vi "Find All COM ports with device Attached.vi"(8 "Error In":errorcluster) -> (0 "Error Out":errorcluster, 3 "List of COM ports with something attached":string[](array[string]))   [LabVIEW 2014]
uses:
  <vilib>/Instr/_visa.llb/VISA Find Search Mode.ctl
panel:
  # "(COM)|?"
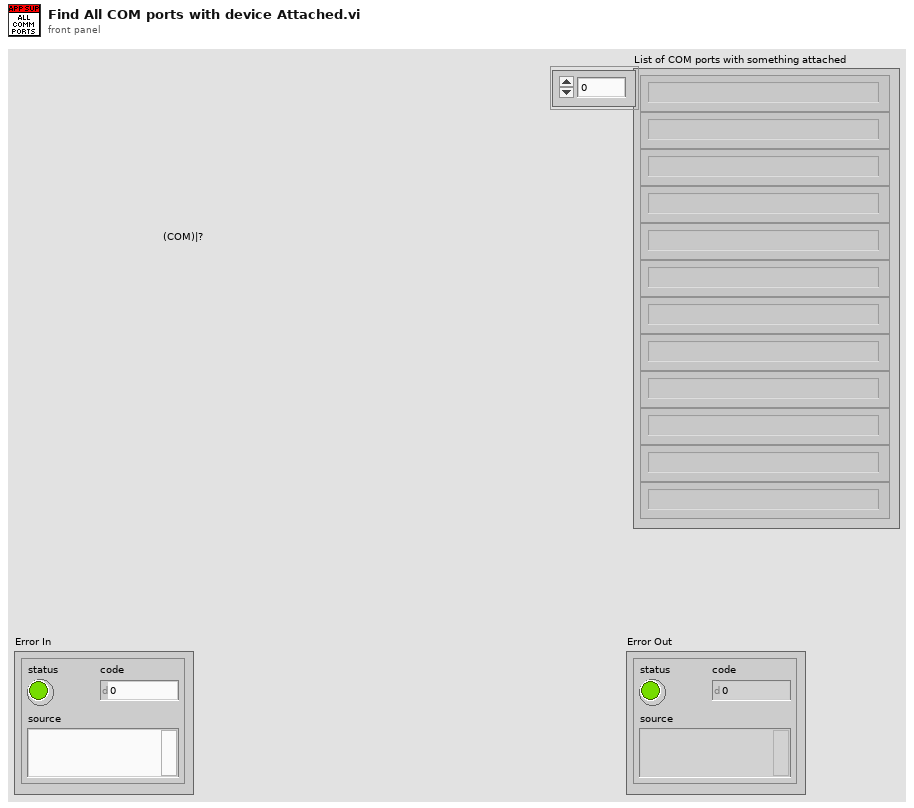
[diagram p1: front panel]
types:
  T1 = typedef "VISA Find Search Mode.ctl" = u32
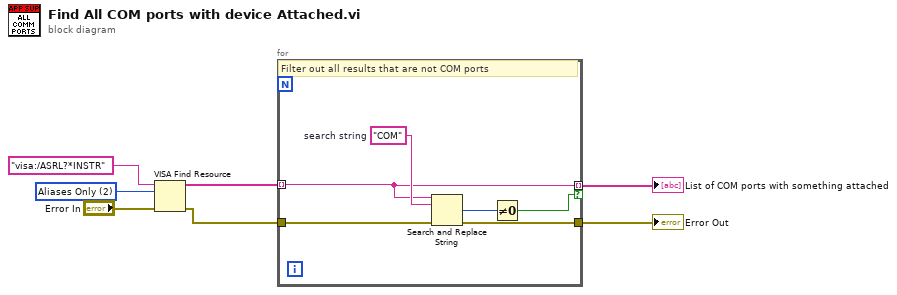
[diagram p0: block diagram]
diagram:
  w7 = T1 2 items=["Canonical Names Only"=0, "Aliases Only"=2, "Include Matching Aliases"=3, "Include All Aliases"=4] ("Search Mode")
  n1 = VISA Find Resource(8:"Error In", 10:w7, 11:"visa:/ASRL?*INSTR" ("expression (\"?*\")")) -> (0:w3:errorcluster, 3:w4:string[])  [unwired: 1 out]
  n2 = for {
    tunnel: w4 -> [w12] mode=indexing
    tunnel: [w12] -> w1 mode=indexing if=w10
    tunnel: w3 -> [w9]
    tunnel: [w8] -> w2
    w13 = "COM"  # search string
    # "Filter out all results that are not COM ports"
    n3 = Search and Replace String(input string=w12, search string=w13, error in=w9) -> (number of replacements=w11:i32, error out=w8:errorcluster)  [unwired: 5 in, 2 out]
    n4 = Not Equal To 0?(x=w11) -> (x != 0?=w10:bool)
  }
  "List of COM ports with something attached" <- w1
  "Error Out" <- w2
